vi "Practica 5 Alejandro Tejada ITIW31.vi"() -> ()   [LabVIEW 2018]
uses:
  <vilib>/express/express analysis/Spectral/Block/exnSpectralBlock spectral measurements RMS poly.vi
  <vilib>/express/express analysis/Spectral/Block/exnSpectralBlock spectral measurements RMS DDT.vi
  <vilib>/express/express analysis/Spectral/XNode/ExpressSpectralMeasurementsBlockNode.xnode
panel:
  out "Waveform Graph 7":dynamicdata(graph)
  out "Comparacion en el dominio del tiempo":dynamicdata(graph)
  out "Waveform Graph 5":dynamicdata(graph)
  out "Waveform Graph 6":dynamicdata(graph)
  out "Waveform Graph 4":dynamicdata(graph)
  out "Waveform Graph 3":dynamicdata(graph)
  out "Waveform Graph 2":dynamicdata(graph)
  out "Waveform Graph":dynamicdata(graph)
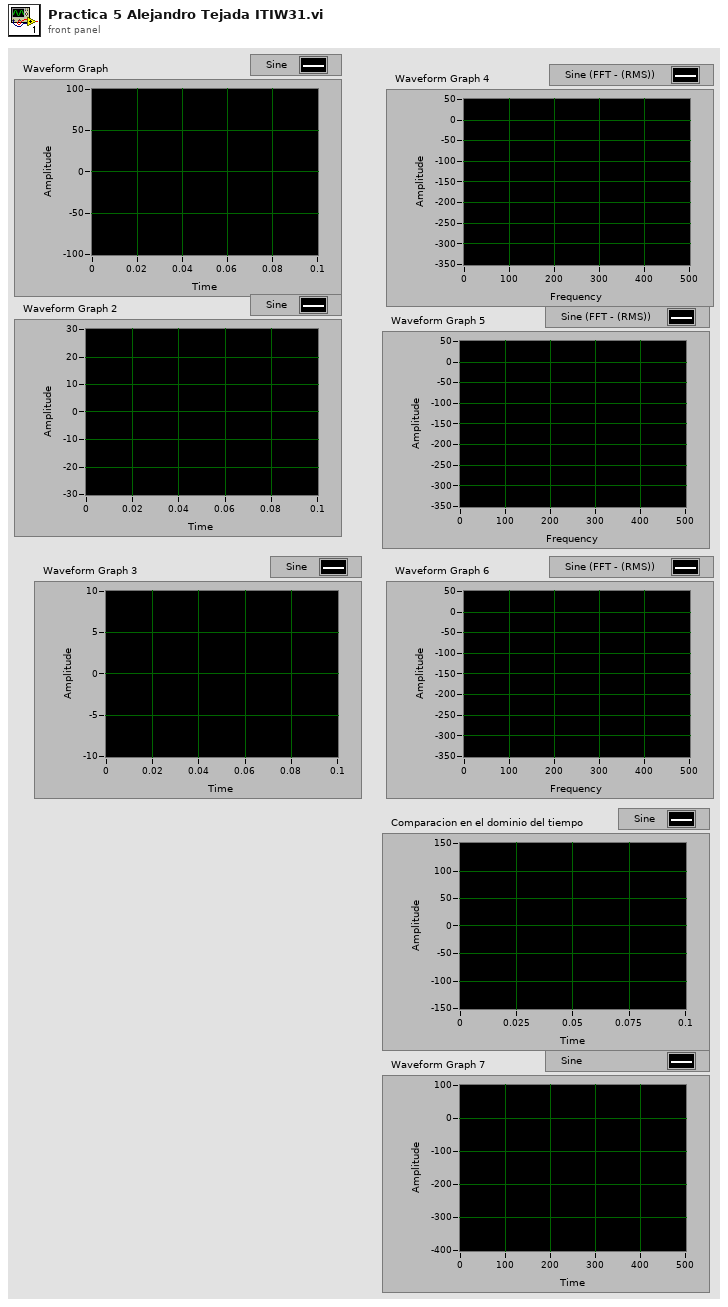
[diagram p1: front panel]
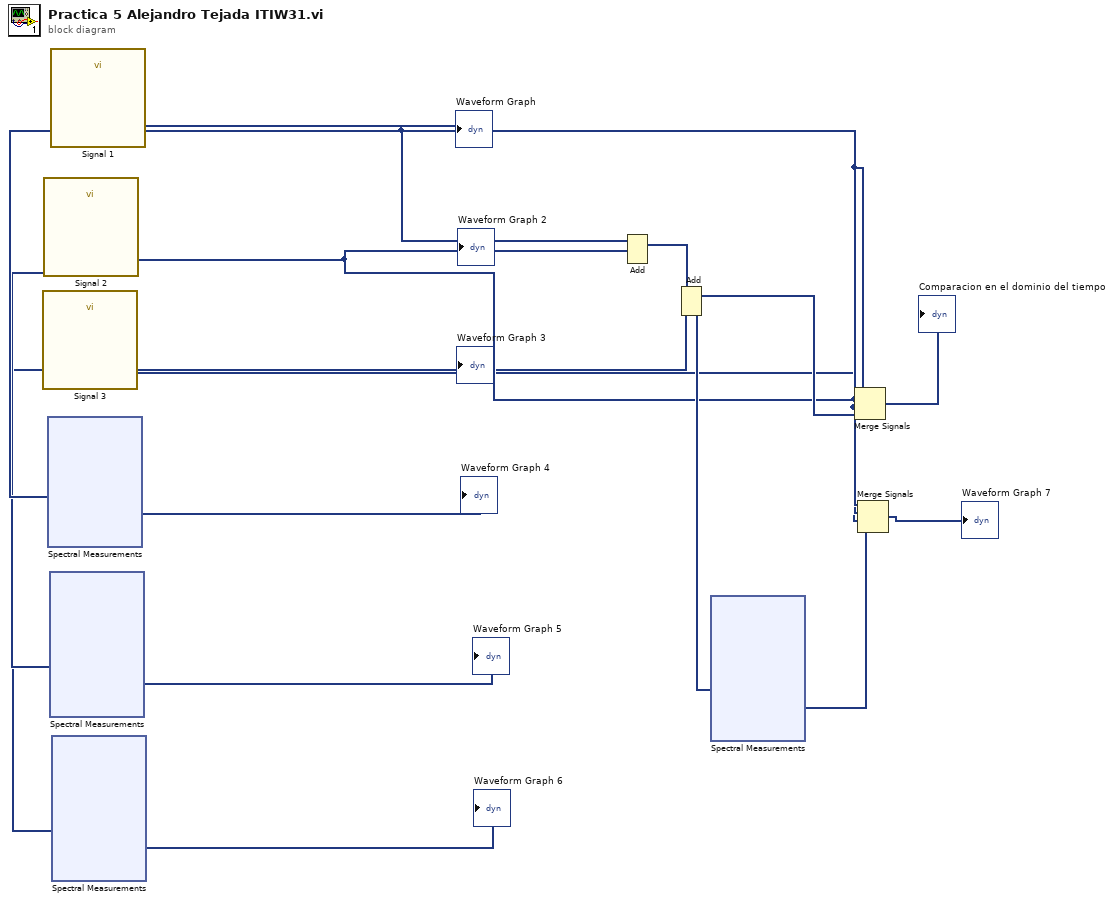
[diagram p0: block diagram]
diagram:
  n1 = call "Signal 3"() -> ("Sine"=w3:dynamicdata)  [unwired: 14 in, 1 out]
  "Waveform Graph 3" <- w3
  n2 = call "Signal 2"() -> ("Sine"=w4:dynamicdata)  [unwired: 14 in, 1 out]
  "Waveform Graph 2" <- w4
  n3 = xnode "Spectral Measurements"("Signals"=w4) -> ("FFT - (RMS)"=→"Waveform Graph 5":dynamicdata)  [unwired: 1 in, 2 out]
  n4 = call "Signal 1"() -> ("Sine"=w5:dynamicdata)  [unwired: 14 in, 1 out]
  "Waveform Graph" <- w5
  n5 = xnode "Spectral Measurements"("Signals"=w5) -> ("FFT - (RMS)"=→"Waveform Graph 4":dynamicdata)  [unwired: 1 in, 2 out]
  n6 = xnode "Spectral Measurements"("Signals"=w3) -> ("FFT - (RMS)"=→"Waveform Graph 6":dynamicdata)  [unwired: 1 in, 2 out]
  n7 = Add(1:w4, 2:w5) -> (0:w8:dynamicdata)  [unwired: 1 in, 1 out]
  n8 = Add(1:w3, 2:w8) -> (0:w6:dynamicdata)  [unwired: 1 in, 1 out]
  n9 = xnode "Spectral Measurements"("Signals"=w6) -> ("FFT - (RMS)"=w2:dynamicdata)  [unwired: 1 in, 2 out]
  n10 = Merge Signals(w5, w4, w3, w6) -> (→"Comparacion en el dominio del tiempo":dynamicdata)
  n11 = Merge Signals(w5, w4, w3, w2) -> (→"Waveform Graph 7":dynamicdata)
